vi "ROS_ParseMsg.vi"(9 "Message Type":string, 11 "msg in":string) -> (1 "data":variant[](array[variant]), 3 "msg out":string)   [LabVIEW 2016]
doc: "Parses a ROS message based on the Message Type. Message Type must be a valid .txt file in the RosMessages directory."
uses:
  std_msgs/subs/parse_bool_scalar.vi
  std_msgs/subs/parse_i8_scalar.vi
  std_msgs/subs/parse_u8_scalar.vi
  std_msgs/subs/parse_i16_scalar.vi
  std_msgs/subs/parse_u16_scalar.vi
  std_msgs/subs/parse_i32_scalar.vi
  std_msgs/subs/parse_u32_scalar.vi
  std_msgs/subs/parse_i64_scalar.vi
  std_msgs/subs/parse_u64_scalar.vi
  std_msgs/subs/parse_float32_scalar.vi
  std_msgs/subs/parse_float64_scalar.vi
  std_msgs/subs/parse_string_scalar.vi
  std_msgs/subs/parse_time_scalar.vi
  std_msgs/subs/parse_duration_scalar.vi
panel:
  out "filenames":string[](array[string])
  out "Data Types":string[](array[string])
  out "Data Names":string[](array[string])
  out "msg def":string
  out "Comments":string[](array[string])
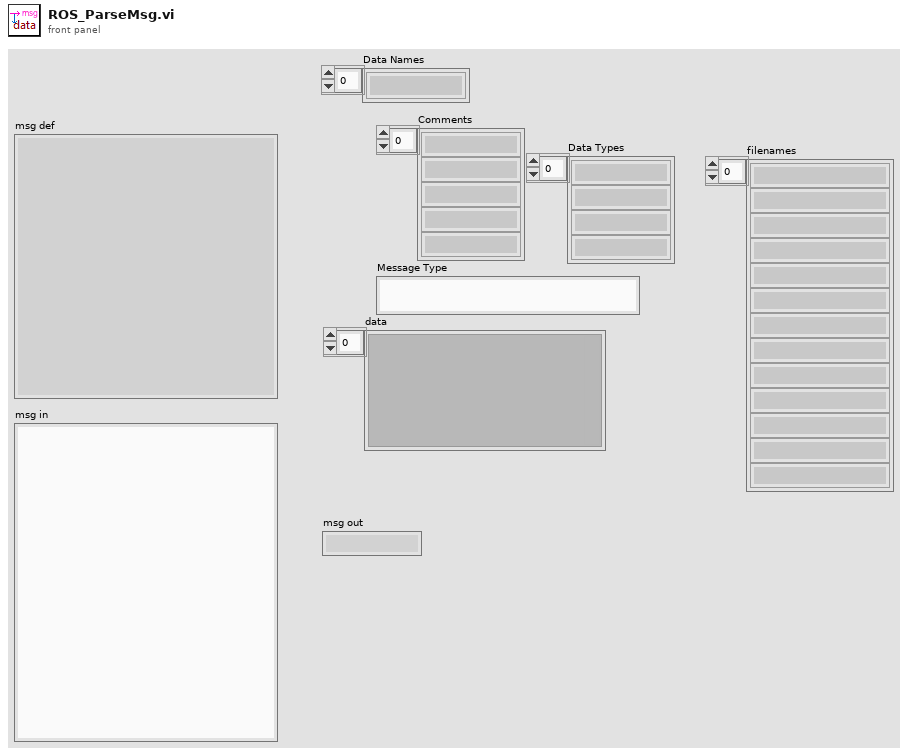
[diagram p1: front panel]
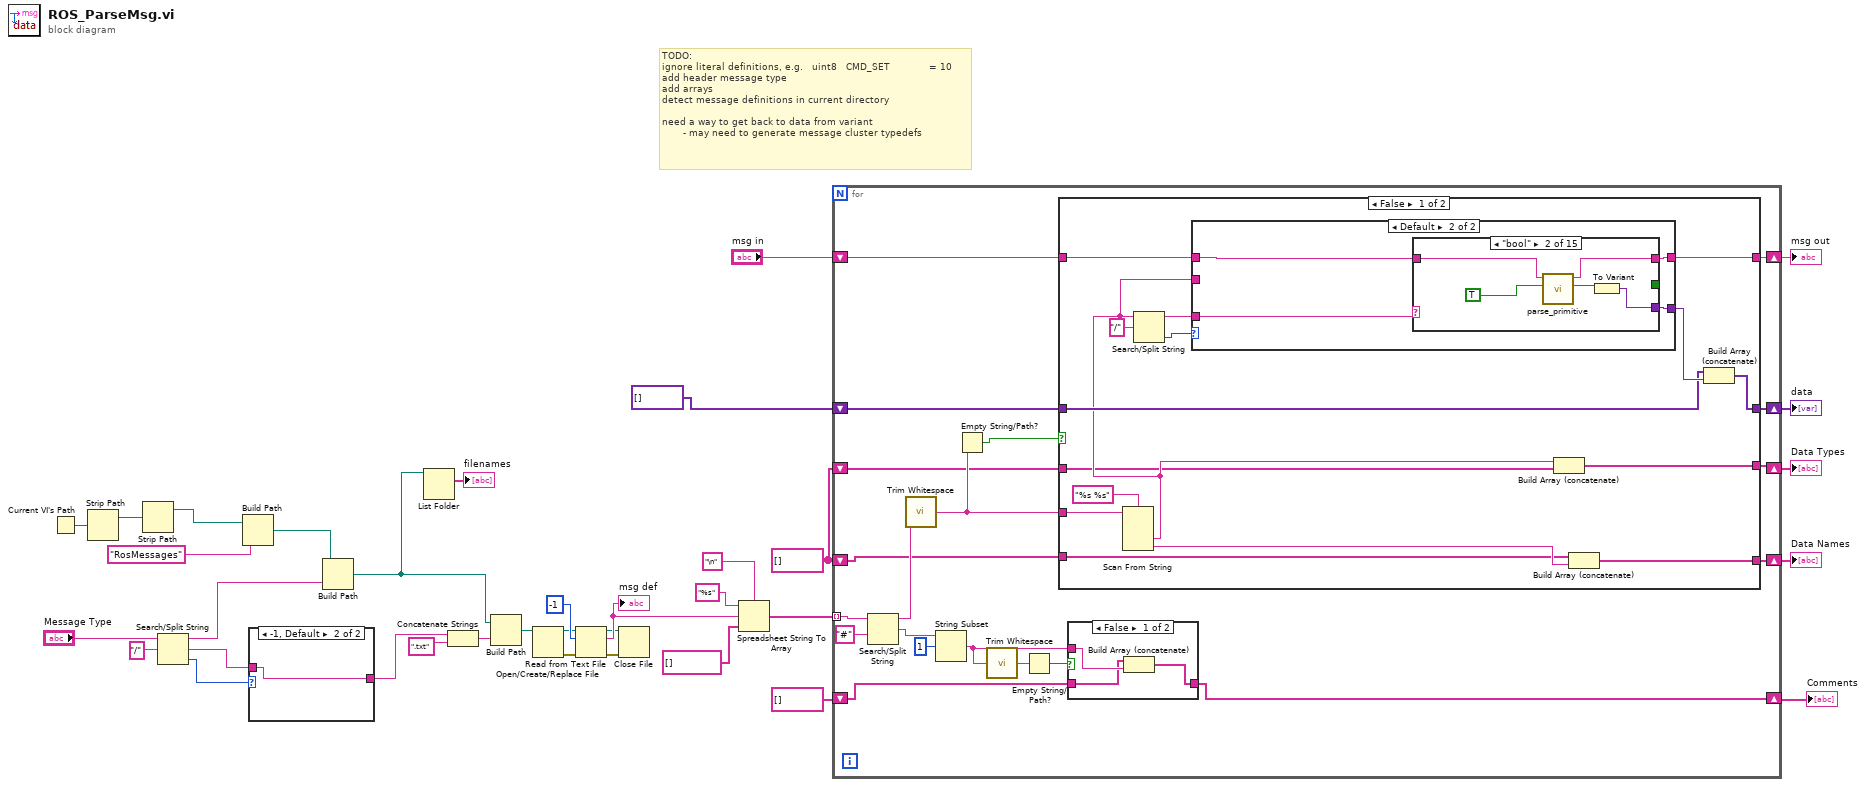
[diagram p0: block diagram]
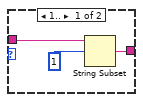
[diagram p2: hidden frame]
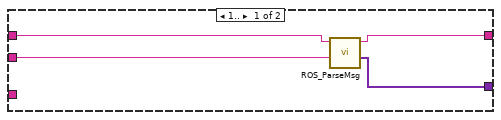
[diagram p3: hidden frame]
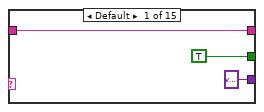
[diagram p4: hidden frame]
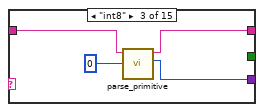
[diagram p5: hidden frame]
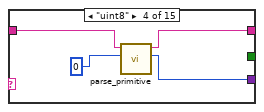
[diagram p6: hidden frame]
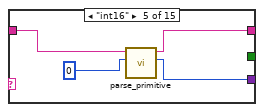
[diagram p7: hidden frame]
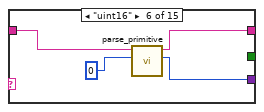
[diagram p8: hidden frame]
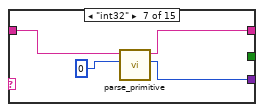
[diagram p9: hidden frame]
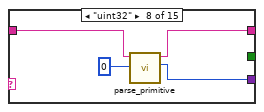
[diagram p10: hidden frame]
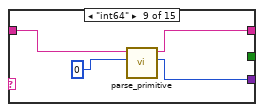
[diagram p11: hidden frame]
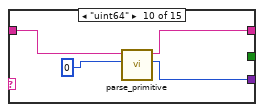
[diagram p12: hidden frame]
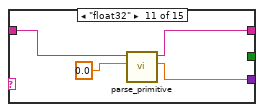
[diagram p13: hidden frame]
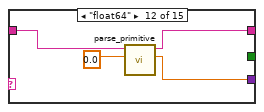
[diagram p14: hidden frame]
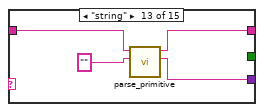
[diagram p15: hidden frame]
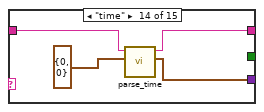
[diagram p16: hidden frame]
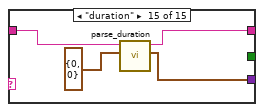
[diagram p17: hidden frame]
diagram:
  w3 = string[] []
  # "TODO:\nignore literal definitions, e.g.   uint8   CMD_SET             = 10\nadd header message type\nadd arrays\ndetect message definitions in current directory\n\nneed a way to get back to data from variant\n       - may need to generate message cluster typedefs"
  n1 = Current VI's Path() -> (path=w21:path)
  n2 = Strip Path(path=w21) -> (stripped path=w20:path)  [unwired: 1 out]
  n3 = Strip Path(path=w20) -> (stripped path=w19:path)  [unwired: 1 out]
  n4 = Search/Split String(string="Message Type", search string/char (-)="/") -> (substring before match=w14:string, match + rest of string=w13:string, offset of match=w4:i32)  [unwired: 1 in]
  n5 = Build Path(base path=w19, name or relative path="RosMessages") -> (appended path=w15:path)
  n6 = case shown="-1, Default" w4 {
    tunnel: w13 -> [w37 w39]
    tunnel: [w36 w39] -> w11
    frame 1.. {
      n7 = String Subset(string=w37, offset (0)=1) -> (substring=w36:string)  [unwired: 1 in]
    }
    frame -1, Default {
    }
  }
  n8 = Build Path(base path=w15, name or relative path=w14) -> (appended path=w2:path)
  n9 = List Folder(path=w2) -> (filenames=→"filenames":string[])  [unwired: 3 in, 3 out]
  n10 = Concatenate Strings(w11, ".txt" ("string")) -> (w12:string)
  n11 = Build Path(base path=w2, name or relative path=w12) -> (appended path=w9:path)
  n12 = Open/Create/Replace File(file path (use dialog)=w9) -> (refnum out=w22:refnum<file>, error out=w23:errorcluster)  [unwired: 5 in, 1 out]
  n13 = Read from Text File(file (use dialog)=w22, count=-1, error in=w23) -> (refnum out=w25:refnum<file>, text=w26:string, error out=w24:errorcluster)  [unwired: 1 in, 1 out]
  "msg def" <- w26
  n14 = Close File(refnum=w25, error in=w24) -> ()  [unwired: 2 out]
  n15 = Spreadsheet String To Array(delimiter (Tab)="\n", format string="%s", spreadsheet string=w26, array type (2D Dbl)=string[] []) -> (array=w32:string[])
  n16 = for {
    tunnel: w32 -> [w58] mode=indexing
    shift-right: [w47] -> w7
    shift-left: variant[] [] -> [w48]
    shift-right: [w51] -> w31
    shift-left: string[] [] -> [w52]
    shift-right: [w49] -> w8
    shift-left: "msg in" -> [w50]
    shift-right: [w43] -> w6
    shift-left: w3 -> [w42]
    shift-right: [w41] -> w5
    shift-left: w3 -> [w40]
    n17 = Search/Split String(string=w58, search string/char (-)="#") -> (substring before match=w46:string, match + rest of string=w57:string)  [unwired: 1 in, 1 out]
    n18 = call "Trim Whitespace.vi"("string"=w46) -> ("trimmed string"=w45:string)  [unwired: 1 in]
    n19 = String Subset(string=w57, offset (0)=1) -> (substring=w53:string)  [unwired: 1 in]
    n20 = Empty String/Path?(string/path=w45) -> (empty?=w44:bool)
    n21 = call "Trim Whitespace.vi"("string"=w53) -> ("trimmed string"=w55:string)  [unwired: 1 in]
    n22 = Empty String/Path?(string/path=w55) -> (empty?=w54:bool)
    n23 = case shown="False" w44 {
      tunnel: w50 -> [w75 w147]
      tunnel: [w74 w147] -> w49
      tunnel: w48 -> [w70 w146]
      tunnel: [w69 w146] -> w47
      tunnel: w45 -> [w72 _]
      tunnel: [w67 w145] -> w43
      tunnel: w42 -> [w66 w145]
      tunnel: [w61 w144] -> w41
      tunnel: w40 -> [w60 w144]
      frame False {
        n24 = Scan From String(format string="%s %s", input string=w72) -> (output 1=w62:string, output 2=w68:string)  [unwired: 4 in, 3 out]
        n25 = Search/Split String(string=w62, search string/char (-)="/") -> (substring before match=w64:string, offset of match=w65:i32)  [unwired: 1 in, 1 out]
        n26 = case shown="Default" w65 {
          tunnel: w75 -> [w79 w83]
          tunnel: [w78 w82] -> w74
          tunnel: [w76 w81] -> w71
          tunnel: w62 -> [w77 _]
          tunnel: w64 -> [_ w80]
          frame 1.. {
            n27 = call "ROS_ParseMsg.vi"("Message Type"=w77, "msg in"=w79) -> ("data"=w76:variant[], "msg out"=w78:string)  [unwired: 8 in]
          }
          frame Default {
            n28 = case shown="\"bool\"" w80 {
              tunnel: w83 -> [w86 w90 w95 w99 w103 w107 w111 w114 w119 w123 w127 w131 w134 w139 w143]
              tunnel: [w86 w89 w94 w97 w102 w105 w109 w113 w118 w122 w125 w129 w133 w137 w142] -> w82
              tunnel: [variant ("Variant") w87 w92 w96 w100 w104 w108 w112 w116 w120 w124 w128 w132 w136 w141] -> w81
              tunnel: [TRUE _ _ _ _ _ _ _ _ _ _ _ _ _ _] -> _
              frame Default {
              }
              frame "bool" {
                n29 = call-poly "parse_primitive.vi"("type"=TRUE, "msg in"=w90) -> ("bool"=w88:bool, "msg out"=w89:string)  [unwired: 3 in, 1 out]
                n30 = To Variant(anything=w88) -> (Variant=w87:variant)
              }
              frame "int8" {
                n31 = call-poly "parse_primitive.vi"("type"=i8 0, "msg in"=w95) -> ("number"=w92:i8, "msg out"=w94:string)  [unwired: 3 in, 1 out]
              }
              frame "uint8" {
                n32 = call-poly "parse_primitive.vi"("type"=u8 0, "msg in"=w99) -> ("number"=w96:u8, "msg out"=w97:string)  [unwired: 3 in, 1 out]
              }
              frame "int16" {
                n33 = call-poly "parse_primitive.vi"("type"=i16 0, "msg in"=w103) -> ("number"=w100:i16, "msg out"=w102:string)  [unwired: 3 in, 1 out]
              }
              frame "uint16" {
                n34 = call-poly "parse_primitive.vi"("type"=u16 0, "msg in"=w107) -> ("number"=w104:u16, "msg out"=w105:string)  [unwired: 3 in, 1 out]
              }
              frame "int32" {
                n35 = call-poly "parse_primitive.vi"("type"=0, "msg in"=w111) -> ("number"=w108:i32, "msg out"=w109:string)  [unwired: 3 in, 1 out]
              }
              frame "uint32" {
                n36 = call-poly "parse_primitive.vi"("type"=u32 0, "msg in"=w114) -> ("number"=w112:u32, "msg out"=w113:string)  [unwired: 3 in, 1 out]
              }
              frame "int64" {
                n37 = call-poly "parse_primitive.vi"("type"=i64 0, "msg in"=w119) -> ("number"=w116:i64, "msg out"=w118:string)  [unwired: 3 in, 1 out]
              }
              frame "uint64" {
                n38 = call-poly "parse_primitive.vi"("type"=u64 0, "msg in"=w123) -> ("number"=w120:u64, "msg out"=w122:string)  [unwired: 3 in, 1 out]
              }
              frame "float32" {
                n39 = call-poly "parse_primitive.vi"("type"=sgl 0.0, "msg in"=w127) -> ("number"=w124:sgl, "msg out"=w125:string)  [unwired: 3 in, 1 out]
              }
              frame "float64" {
                n40 = call-poly "parse_primitive.vi"("type"=0.0, "msg in"=w131) -> ("number"=w128:dbl, "msg out"=w129:string)  [unwired: 3 in, 1 out]
              }
              frame "string" {
                n41 = call-poly "parse_primitive.vi"("type"="" ("delimiter (Tab)"), "msg in"=w134) -> ("string"=w132:string, "msg out"=w133:string)  [unwired: 3 in, 1 out]
              }
              frame "time" {
                n42 = call-poly "parse_time.vi"("type"=cluster{"secs":i32, "nsecs":i32} {"secs"=0, "nsecs"=0}, "msg in"=w139) -> ("Time"=w136:cluster{"secs":i32, "nsecs":i32}, "msg out"=w137:string)  [unwired: 3 in, 1 out]
              }
              frame "duration" {
                n43 = call-poly "parse_duration.vi"("type"=cluster{"secs":i32, "nsecs":i32} {"secs"=0, "nsecs"=0}, "msg in"=w143) -> ("Duration"=w141:cluster{"secs":i32, "nsecs":i32}, "msg out"=w142:string)  [unwired: 3 in, 1 out]
              }
            }
          }
        }
        n44 = Build Array (concatenate)(w62, w60) -> (w61:string[])
        n45 = Build Array (concatenate)(w66, w68) -> (w67:string[])
        n46 = Build Array (concatenate)(w70, w71) -> (w69:variant[])
      }
      frame True {
      }
    }
    n47 = case shown="False" w54 {
      tunnel: w53 -> [w150 _]
      tunnel: w52 -> [w149 w151]
      tunnel: [w148 w151] -> w51
      frame False {
        n48 = Build Array (concatenate)(w149, w150) -> (w148:string[])
      }
      frame True {
      }
    }
  }
  "Comments" <- w31
  "msg out" <- w8
  "data" <- w7
  "Data Names" <- w6
  "Data Types" <- w5
